vi "Test - Engine.vi"(8 "error in (no error)":errorcluster) -> (0 "error out":errorcluster)   [LabVIEW 2017]
uses:
  Controls/Test - Driver control.ctl
  Controls/RT- Queue States.ctl
  <vilib>/Utility/file.llb/Read Delimited Spreadsheet (string).vi
  Test - Step config.ctl
  Test - Message cluster.ctl
  SubVIs/SubVI - Global.vi
  <vilib>/Platform/TimedLoop/XDataNode/XDataNode.xnode
  <vilib>/Platform/TimedLoop/XDataNode/nitl_modes.ctl
  <vilib>/Platform/TimedLoop/XDataNode/XDNodeRunTimeDep.lvlib
  <vilib>/Platform/TimedLoop/XDataNode/wakeup.ctl
  <vilib>/Platform/TimedLoop/XDataNode/timing_clust.ctl
  Test - Step Result.ctl
  Controls/RT- Get Set.ctl
  DataLog/Datalog -Driver Control.ctl
  DAQ/DAQ -Driver Control.ctl
  Controls/TCP - Driver Control.ctl
  Controls/TCP - Signal Names.ctl
  Controls/TCP - Signals.ctl
  Controls/Dyno Config Driver.ctl
  SubVIs/Get - Set.ctl
panel:
  out "appended array":T1[](array[typedef])
  out "Waveform Chart":dbl(graph)
  out "Results":T2[](array[typedef])
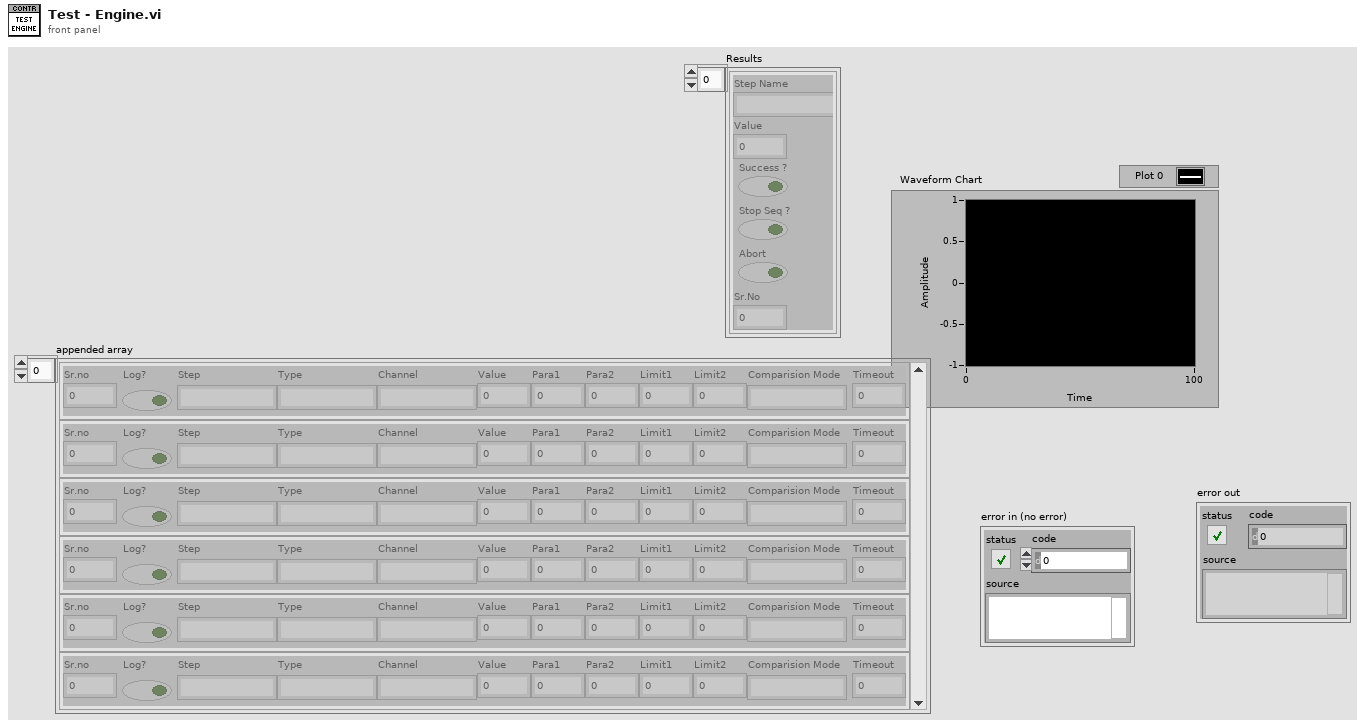
[diagram p1: front panel]
types:
  T1 = typedef "Test - Step config.ctl" = cluster{"Sr.no":i32, "Log?":bool, "Step":string, "Type":string, "Channel":string, "Value":dbl, "Para1":dbl, "Para2":dbl, "Limit1":dbl, "Limit2":dbl, "Comparision Mode":string, "Timeout":dbl}
  T2 = typedef "Test - Step Result.ctl" = cluster{"Step Name":string, "Value":dbl, "Success ?":bool, "Stop Seq ?":bool, "Abort":bool, "Sr.No":i32}
  T3 = typedef "Test - Message cluster.ctl" = cluster{"Preslip Sequence":T1[], "Step No":i32, "Step Value":T1, "Slip Parameter":T1[], "Slip Timer":dbl, "Postslip Sequence":T1[], "Postslip ?":bool, "Step Result":T2}
  T4 = typedef "Test - Driver control.ctl" = enum16{"Init", "Load Sequence File", "Test Running", "Index Step", "Execute Step", "Send Results", "Sequence Complete", "Sequence Aborted", "Stop Sequence Triggered", "Update Manual Values", "Start Aux Logging", "Stop Aux Logging", "Change Dyno Selection", "Reset Emergency Fault", "Get Dyno Config", "Exit"}
  T5 = typedef "RT- Queue States.ctl" = enum16{"Initialize", "Enqueue", "Enqueue Priority", "Dequeue", "Flush", "Destroy"}
  T6 = typedef "Dyno Config Driver.ctl" = enum16{"Read File", "Set", "Get", "Write File", "Set Temp Value"}
  T7 = typedef "Get - Set.ctl" = enum16{"SET", "GET", "Derived"}
  T8 = typedef "TCP - Driver Control.ctl" = enum16{"Download Config Files", "Test Started", "Test Running", "Update Sensor Data", "Test Complete"}
  T9 = typedef "TCP - Signal Names.ctl" = enum16{"Test Running", "Update Sensor Data", "Start Test", "Test Started", "Sequence Complete", "Seuence Aborted", "Abort Test", "Test Settings Updated", "Log Path", "Start Aux Logging", "Stop Aux Logging", "Reset Emergency", "Copy Log File", "Generate Alarm", "Download Files", "Send Test Details"}
  T10 = typedef "TCP - Signals.ctl" = cluster{"Signal":T9, "Value":bool, "Data":variant}
  T11 = typedef "RT- Get Set.ctl" = enum16{"Reset", "Get", "Set"}
  T12 = typedef "Datalog -Driver Control.ctl" = enum16{"Timeout", "Init", "Create Date Folder", "Create File", "Log Data", "Close File", "Update Fileinfo", "Download Files from Windows", "Exit"}
  T13 = typedef "DAQ -Driver Control.ctl" = enum16{"Timeout", "Init", "Config FPGA", "Start Acquisition", "Read Data", "Stop Acquisition", "Flush Queue", "Exit"}
  T14 = typedef "XDNodeRunTimeDep.lvlib/timing_clust.ctl" = cluster{"Expected End [f-1]":u64, "Actual End [f-1]":u64, "Finished Late? [f-1]":bool, "Expected End [i-1]":u64, "Actual End [i-1]":u64, "Finished Late? [i-1]":bool, "Expected Start [i]":u64, "Actual Start [i]":u64, "Expected Start [f]":u64, "Actual Start [f]":u64, "Source Name":string, "Structure Name":string, "Period":i64, "Deadline":i64, "Offset":i64, "Start":i64, "Priority":i32, "Timeout":i32, "Mode":T15, "Wakeup Reason":T16, "Error":errorcluster, "Source Type":string, "Secondary Source Type":string, "Global End Time":u64, "Global Start Time":u64, "Frame Duration":u64, "Iteration Duration":u64, "Assigned CPU":i32, "I/O Scan Engine Mode":u32}
  T15 = typedef "XDNodeRunTimeDep.lvlib/nitl_modes.ctl" = enum32{"No Change", "Process missed periods, maintain original phase", "Discard missed periods, maintain original phase", "Process missed periods, ignore original phase", "Discard missed periods, ignore original phase"}
  T16 = typedef "XDNodeRunTimeDep.lvlib/wakeup.ctl" = enum32{"Normal", "Aborted", "Asynchronous wakeup", "Timing source error", "Timed loop error", "Timeout"}
  T17 = typedef "TCP - Driver Control.ctl" = enum16{"Test Settings", "Boolean Commands", "Test Results"}
  T18 = typedef "TCP - Signal Names.ctl" = enum16{"Start Test", "Test Started", "Sequence Complete", "Seuence Aborted", "Abort Test", "Test Settings Updated", "Log Path", "Update Manual Values", "Start Aux Logging", "Aux Log Started", "Stop Aux Logging", "Aux Log Stopped", "Set Dyno Config", "Get PID Values", "Reset Emergency", "Copy Log File", "Download Files"}
  T19 = cluster{"proportional gain (Kc)":dbl, "integral time (Ti, min)":dbl, "derivative time (Td, min)":dbl}
  T20 = typedef "RT- Dyno Parameters.ctl" = cluster{"PID gains":cluster{"proportional gain (Kc)":dbl, "integral time (Ti, min)":dbl, "derivative time (Td, min)":dbl}, "Channel No":i32, "Dyno Type":string}
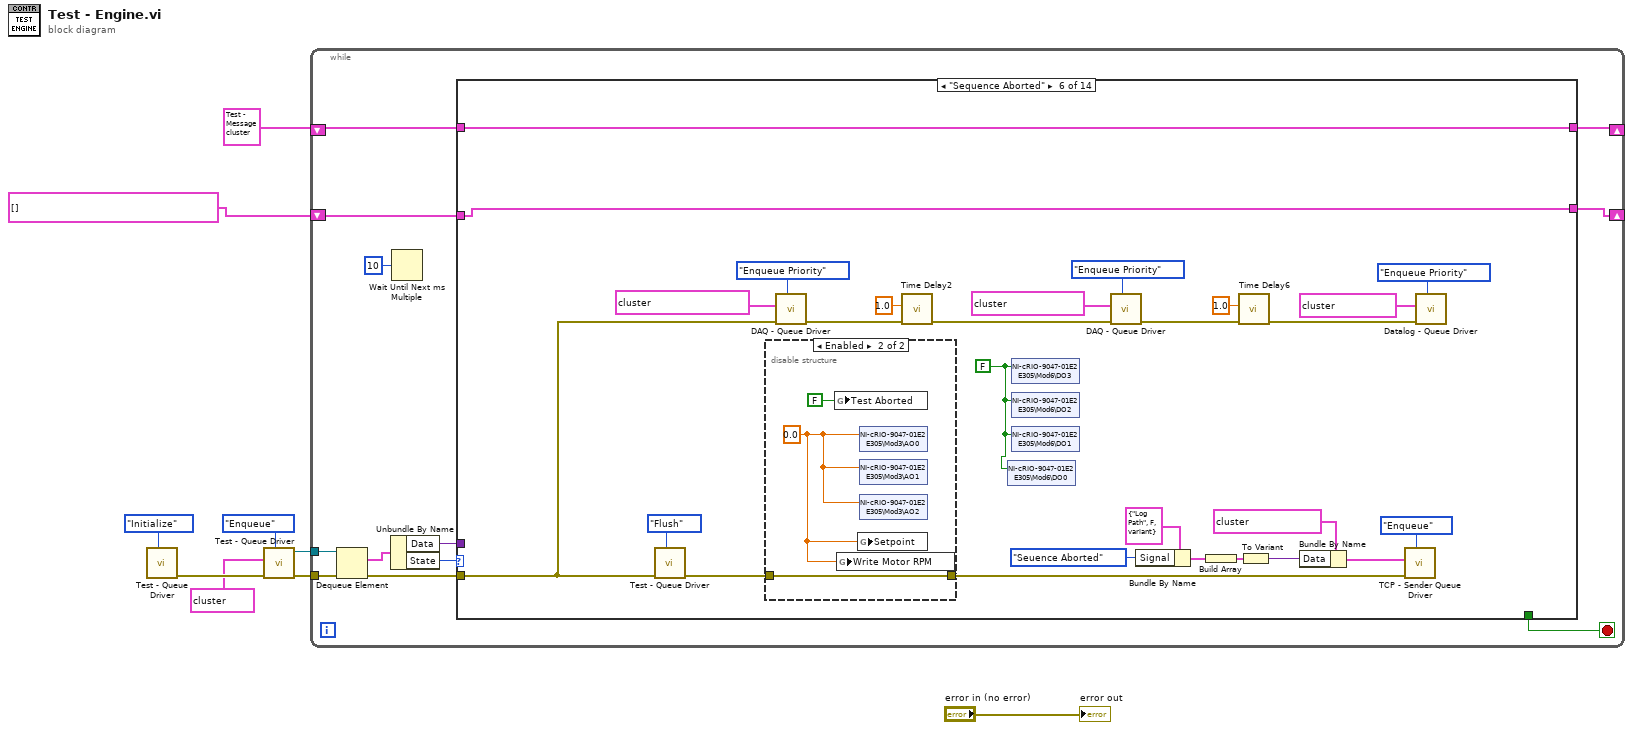
[diagram p0: block diagram]
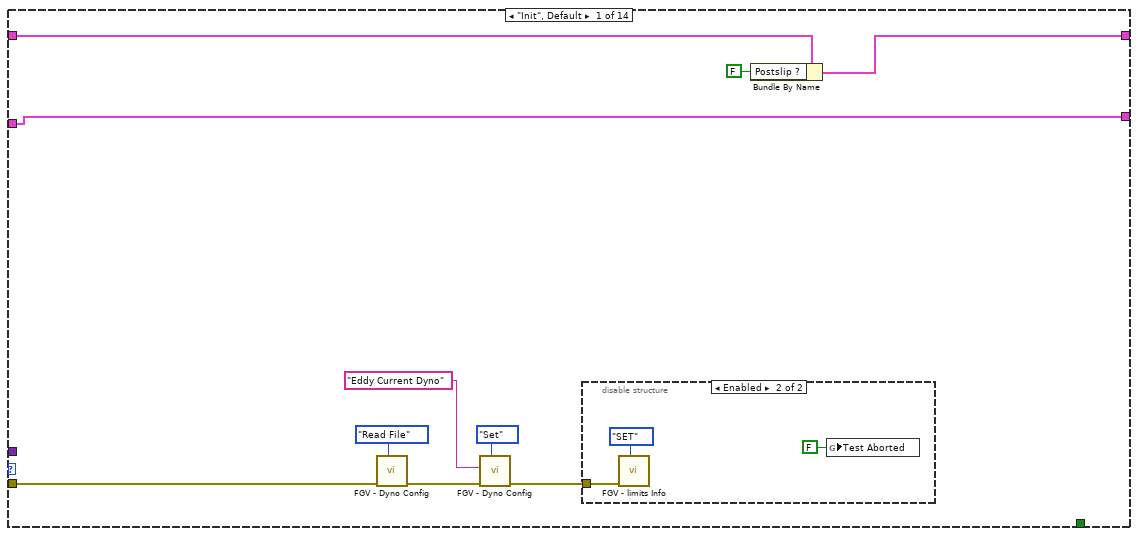
[diagram p2: hidden frame]
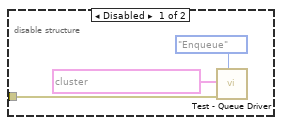
[diagram p3: hidden frame]
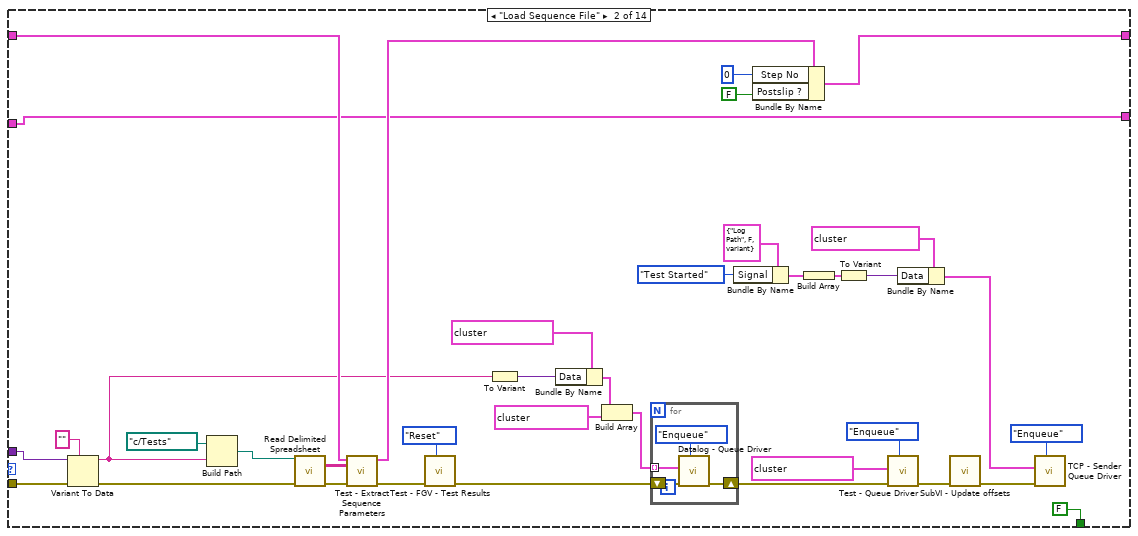
[diagram p4: hidden frame]
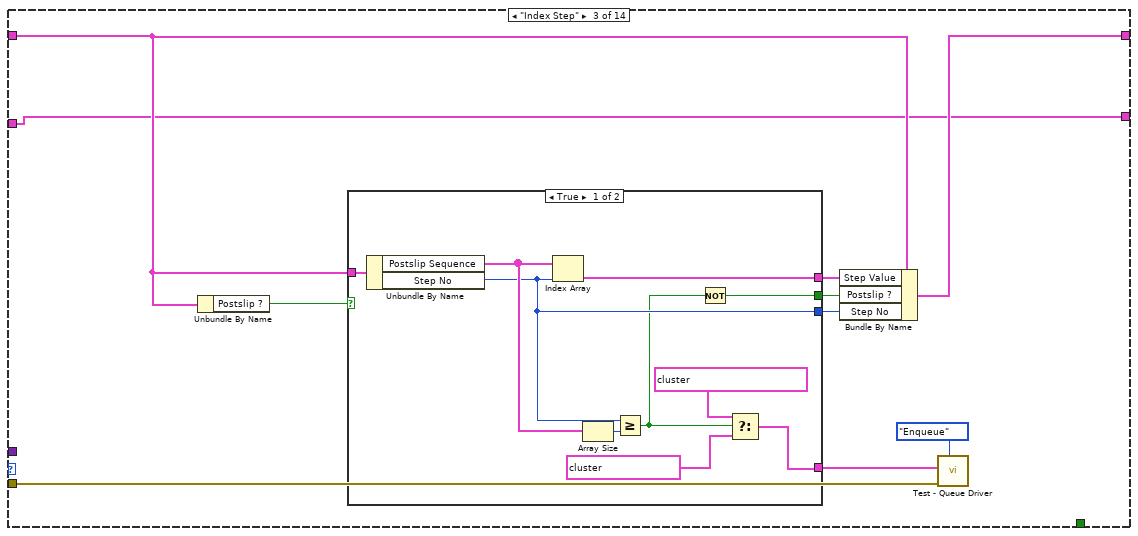
[diagram p5: hidden frame]
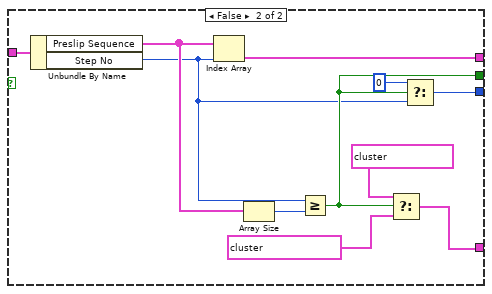
[diagram p6: hidden frame]
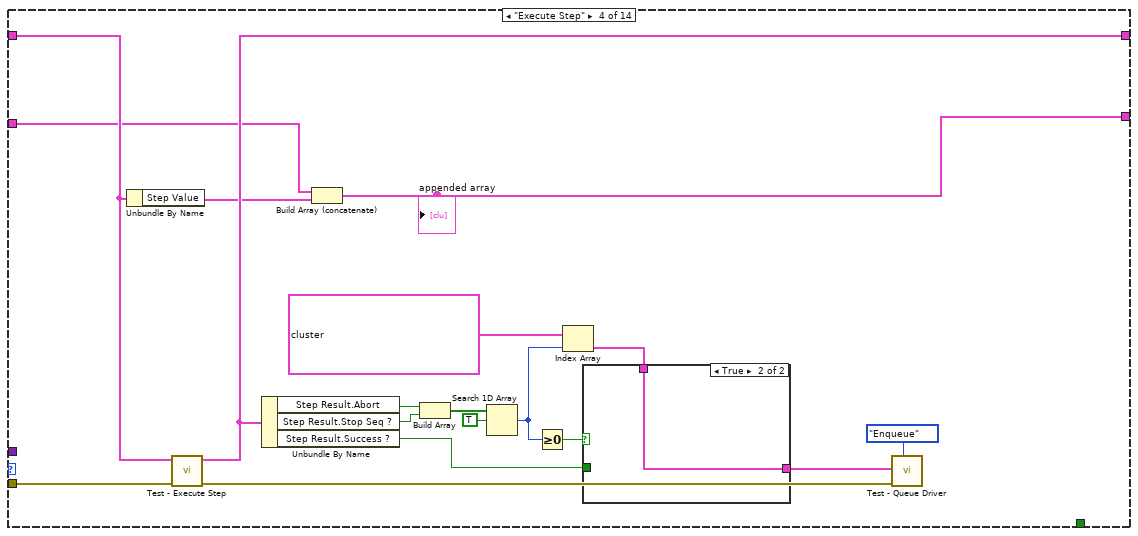
[diagram p7: hidden frame]
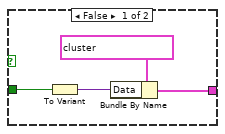
[diagram p8: hidden frame]
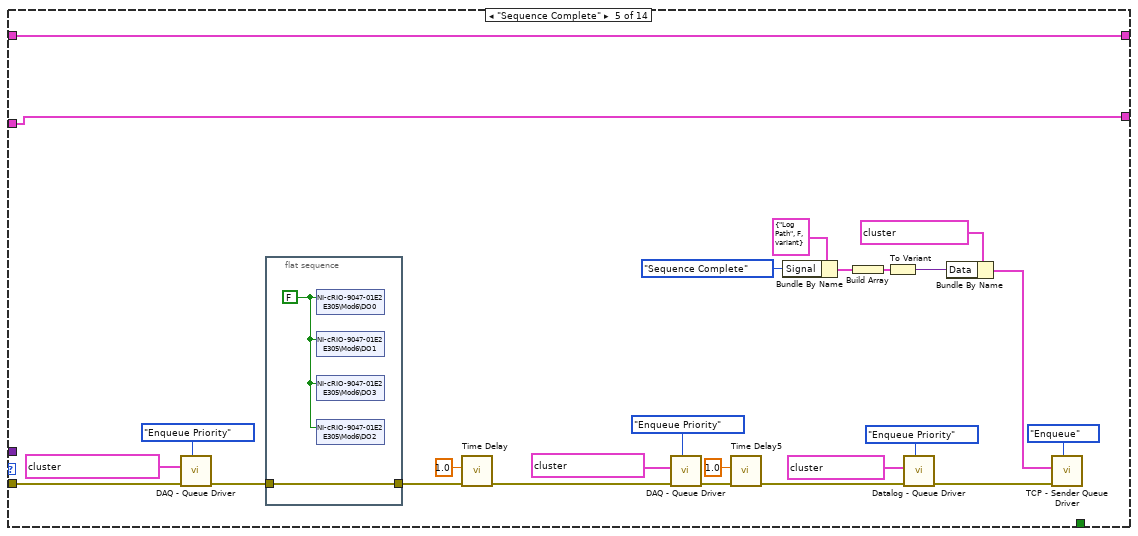
[diagram p9: hidden frame]
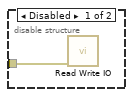
[diagram p10: hidden frame]
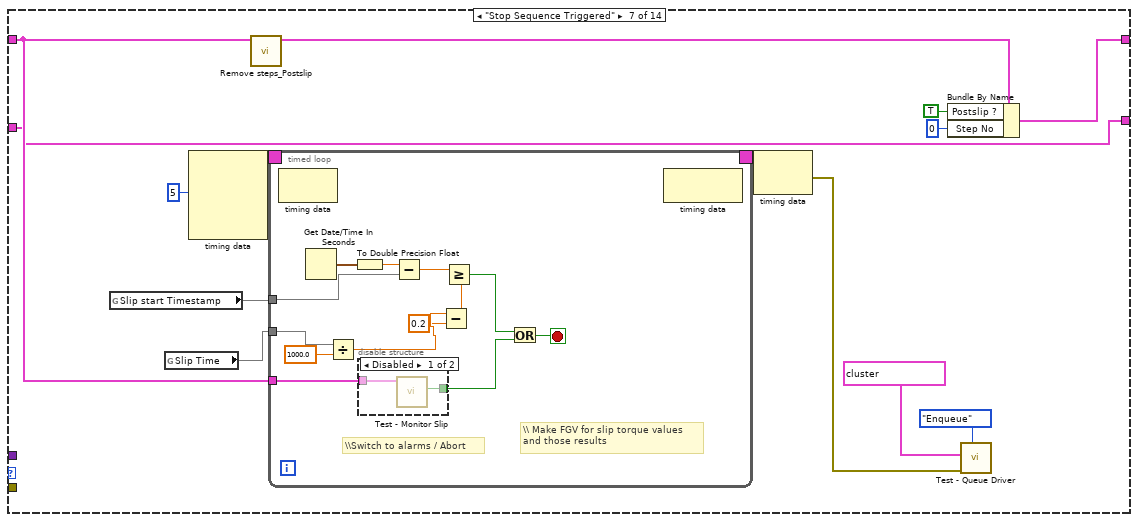
[diagram p11: hidden frame]
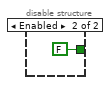
[diagram p12: hidden frame]
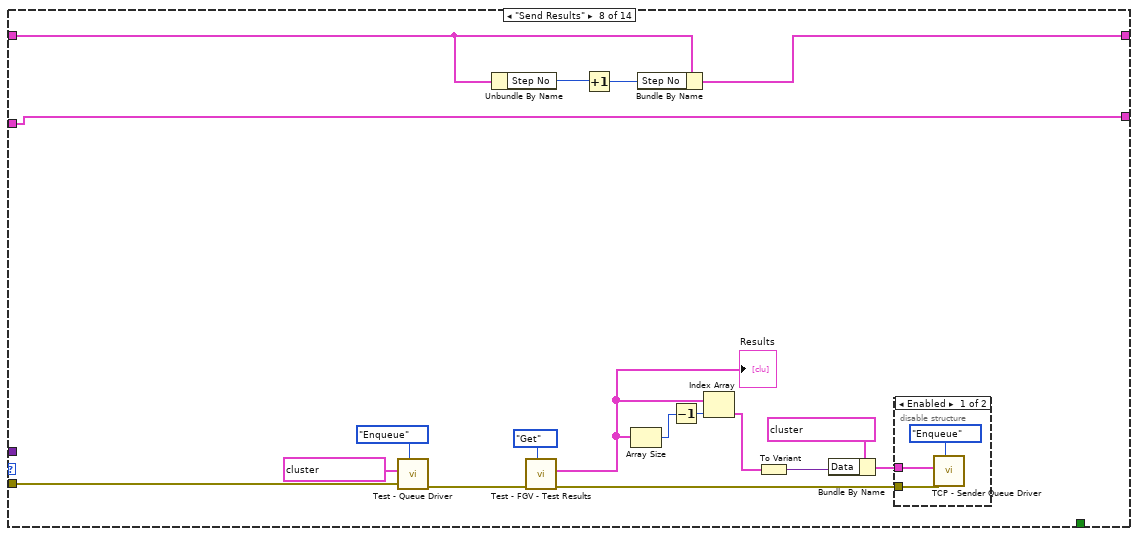
[diagram p13: hidden frame]
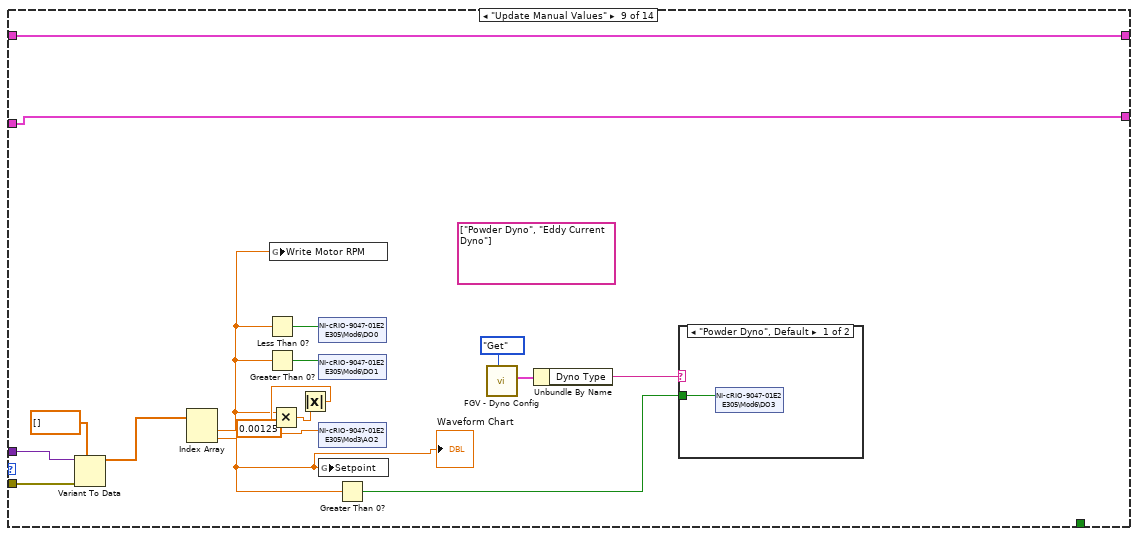
[diagram p15: hidden frame]
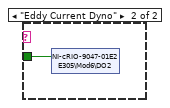
[diagram p16: hidden frame]
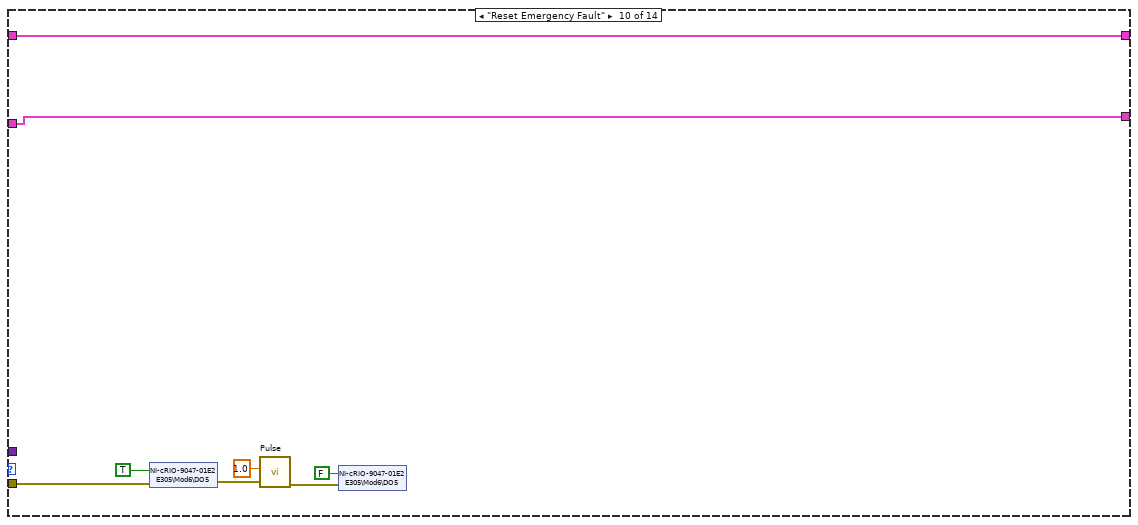
[diagram p17: hidden frame]
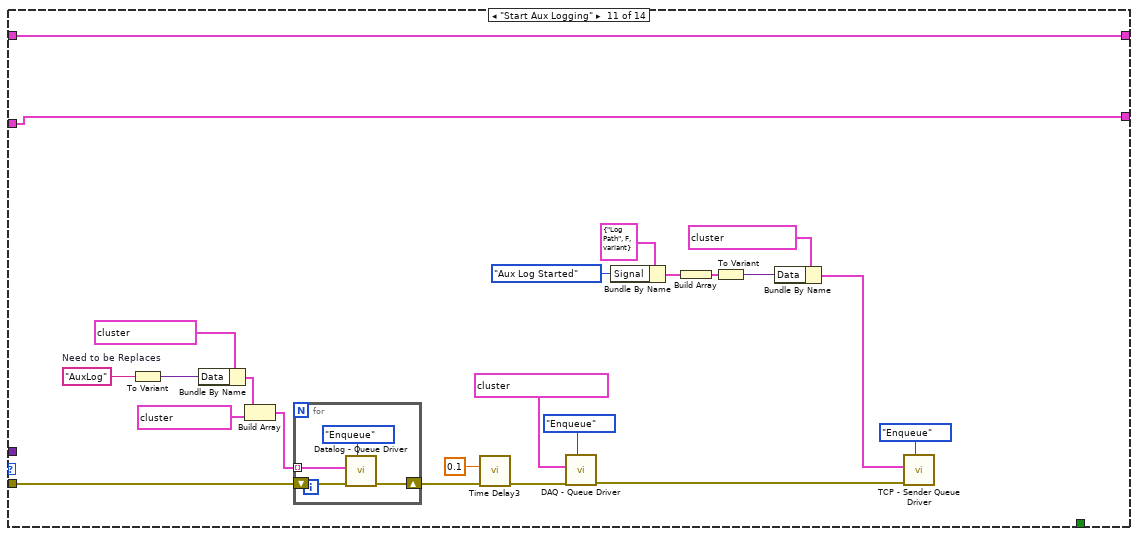
[diagram p18: hidden frame]
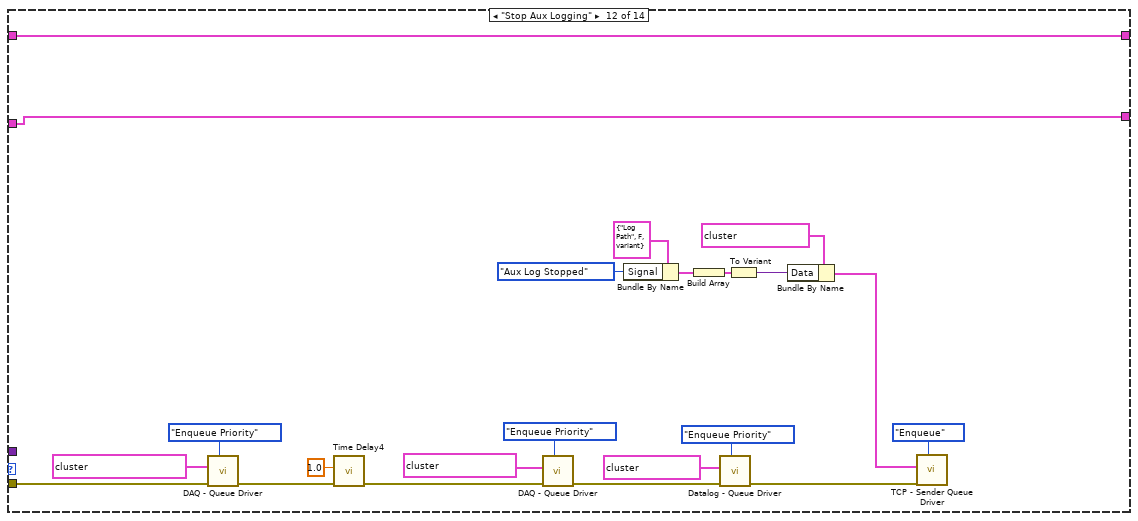
[diagram p19: hidden frame]
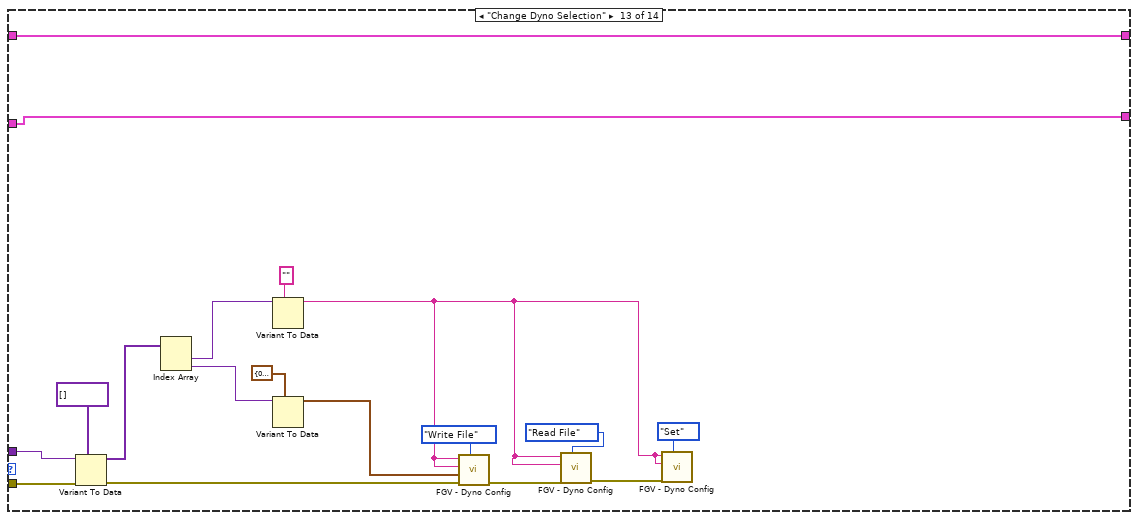
[diagram p20: hidden frame]
diagram:
  n1 = call "Test - Queue Driver.vi"("Cases"=RT-_Queue_States."Initialize") -> ("error out"=w7:errorcluster)  [unwired: 8 in, 2 out]
  n2 = call "Test - Queue Driver.vi"("Cases"=RT-_Queue_States."Enqueue", "error in (no error)"=w7, "Element In"=cluster{"Data":variant, "State":T4} {"Data"=variant, "State"=enum."Init"}) -> ("error out"=w5:errorcluster, "queue out"=w4:refnum<queue>)  [unwired: 6 in, 1 out]
  n3 = while {
    tunnel: w5 -> [w21]
    tunnel: w4 -> [w20]
    shift-right: [w13] -> _
    shift-left: T3 {"Preslip Sequence"=[], "Step No"=0, "Step Value"={"Sr.no"=0, "Log?"=FALSE, "Step"="", "Type"="", "Channel"="", "Value"=0.0, "Para1"=0.0, "Para2"=0.0, "Limit1"=0.0, "Limit2"=0.0, "Comparision Mode"="", "Timeout"=0.0}, "Slip Parameter"=[], "Slip Timer"=0.0, "Postslip Sequence"=[], "Postslip ?"=FALSE, "Step Result"={"Step Name"="", "Value"=0.0, "Success ?"=TRUE, "Stop Seq ?"=TRUE, "Abort"=TRUE, "Sr.No"=0}} -> [w12]
    shift-right: [w10] -> _
    shift-left: T1[] [] ("element") -> [w11]
    stop <- w14 stop-if-true
    n4 = Dequeue Element(queue=w20, error in (no error)=w21) -> (element=w19:cluster{"Data":variant, "State":T4}, error out=w18:errorcluster)  [unwired: 1 in, 2 out]
    n5 = Unbundle By Name(w19) -> ("Data"=w16:variant, "State"=w17:T4)
    n6 = Wait Until Next ms Multiple(millisecond multiple=u32 10) -> ()  [unwired: 1 out]
    n7 = case shown="\"Sequence Aborted\"" w17 {
      tunnel: w18 -> [w27 w53 w85 w127 w152 w175 _ w239 w264 w269 w291 w319 w340 w360]
      tunnel: w16 -> [_ w55 _ _ _ _ _ _ w263 _ _ _ w339 w358]
      tunnel: [_ FALSE _ _ _ _ _ _ _ _ _ _ _ _] -> w14
      tunnel: w12 -> [w30 w73 w83 w113 w157 w186 w193 w243 w265 w275 w298 w324 w342 w363]
      tunnel: [w29 w66 w87 w117 w157 w186 w199 w242 w265 w275 w298 w324 w342 w363] -> w13
      tunnel: w11 -> [w22 w38 w79 w111 w135 w161 w191 w228 w249 w268 w276 w303 w325 w343]
      tunnel: [w22 w38 w79 w110 w135 w161 w191 w228 w249 w268 w276 w303 w325 w343] -> w10
      frame "Init", Default {
        n8 = call "FGV - Dyno Config.vi"("Control"=Dyno_Config_Driver."Read File", "error in (no error)"=w27) -> ("error out"=w25:errorcluster)  [unwired: 8 in, 1 out]
        n9 = call "FGV - Dyno Config.vi"("Control"=Dyno_Config_Driver."Set", "error in (no error)"=w25, "Dyno"="Eddy Current Dyno") -> ("error out"=w24:errorcluster)  [unwired: 7 in, 1 out]
        n10 = disable-structure shown="Enabled" {
          disable-tunnel: w24 -> [w32 w35]
          frame Disabled {
            n11 = call "Test - Queue Driver.vi"("Cases"=RT-_Queue_States."Enqueue", "error in (no error)"=w32, "Element In"=cluster{"Data":variant, "State":T4} {"Data"=variant, "State"=enum."Load Sequence File"}) -> ()  [unwired: 6 in, 3 out]
          }
          frame Enabled {
            n12 = call "FGV - limits Info.vi"("GET/SET"=Get_-_Set."SET", "error in (no error)"=w35) -> ()  [unwired: 8 in, 2 out]
            n13 = global write "SubVI - Global.vi" "Test Aborted"(FALSE ("Test Aborted")) -> ()
          }
        }
        n14 = Bundle By Name(cluster=w30, "Postslip ?"=FALSE) -> (w29:T3)
      }
      frame "Load Sequence File" {
        n15 = Variant To Data(error in=w53, type="", Variant=w55) -> (data=w41:string, error out=w52:errorcluster)
        n16 = Build Path(base path=path "c:/Tests" ("file path (dialog if empty)"), name or relative path=w41) -> (appended path=w50:path)
        n17 = call-poly <vilib>:"Read Delimited Spreadsheet.vi"("file path (dialog if empty)"=w50, "error in (no error)"=w52) -> ("all rows"=w72:string[][], "error out"=w71:errorcluster)  [unwired: 8 in, 4 out]
        n18 = call "Test - Extract Sequence Parameters.vi"("error in (no error)"=w71, "Sequence Data"=w72, "Cluster in"=w73) -> ("error out"=w57:errorcluster, "output cluster"=w67:T3)  [unwired: 7 in]
        n19 = call "Test - FGV - Test Results.vi"("Get/Set"=RT-_Get_Set."Reset", "error in (no error)"=w57) -> ("error out"=w56:errorcluster)  [unwired: 8 in, 1 out]
        n20 = To Variant(anything=w41) -> (Variant=w64:variant)
        n21 = Bundle By Name(cluster=cluster{"Data":variant, "State":T12} {"Data"=variant, "State"=enum."Create File"} ("Element In"), "Data"=w64) -> (w60:cluster{"Data":variant, "State":T12})
        n22 = Build Array(w60, cluster{"Data":variant, "State":T12} {"Data"=variant, "State"=enum."Log Data"} ("element")) -> (w59:cluster{"Data":variant, "State":T12}[])
        n23 = for {
          tunnel: w59 -> [w75] mode=indexing
          shift-right: [w76] -> w62
          shift-left: w56 -> [w77]
          n24 = call "Datalog - Queue Driver.vi"("Cases"=RT-_Queue_States."Enqueue", "error in (no error)"=w77, "Element In"=w75) -> ("error out"=w76:errorcluster)  [unwired: 6 in, 2 out]
        }
        n25 = Bundle By Name(cluster=T10 {"Signal"=enum."Log Path", "Value"=FALSE, "Data"=variant}, "Signal"=TCP_-_Signal_Names."Test Started") -> (w46:T10)
        n26 = Bundle By Name(cluster=w67, "Step No"=0, "Postslip ?"=FALSE) -> (w66:T3)
        n27 = Build Array(w46) -> (w44:T10[])
        n28 = To Variant(anything=w44) -> (Variant=w43:variant)
        n29 = call "Test - Queue Driver.vi"("Cases"=RT-_Queue_States."Enqueue", "error in (no error)"=w62, "Element In"=cluster{"Data":variant, "State":T4} {"Data"=variant, "State"=enum."Index Step"}) -> ("error out"=w40:errorcluster)  [unwired: 6 in, 2 out]
        n30 = Bundle By Name(cluster=cluster{"Data":variant, "State":T8} {"Data"=variant, "State"=enum."Test Started"} ("Element In"), "Data"=w43) -> (w42:cluster{"Data":variant, "State":T8})
        n31 = call "SubVI - Update offsets.vi"("error in (no error)"=w40) -> ("error out"=w39:errorcluster)  [unwired: 10 in]
        n32 = call "TCP - Sender Queue Driver.vi"("Cases"=RT-_Queue_States."Enqueue", "error in (no error)"=w39, "Element In"=w42) -> ()  [unwired: 6 in, 3 out]
      }
      frame "Index Step" {
        n33 = Unbundle By Name(w83) -> ("Postslip ?"=w82:bool)
        n34 = case shown="True" w82 {
          tunnel: [w98 w103] -> w88
          tunnel: [w94 w106] -> w84
          tunnel: w83 -> [w93 w105]
          tunnel: [w89 w102] -> w81
          tunnel: [w91 w99] -> w80
          frame True {
            n35 = Unbundle By Name(w93) -> ("Postslip Sequence"=w97:T1[], "Step No"=w91:i32)
            n36 = Index Array(array=w97, index=w91) -> (element=w98:T1)
            n37 = Array Size(array=w97) -> (size(s)=w92:i32)
            n38 = Greater Or Equal?(x=w91, y=w92) -> (x >= y?=w90:bool)
            n39 = Not(x=w90) -> (.not. x?=w89:bool)
            n40 = Select(t=cluster{"Data":variant, "State":T4} {"Data"=variant, "State"=enum."Sequence Complete"} ("Element In"), s=w90, f=cluster{"Data":variant, "State":T4} {"Data"=variant, "State"=enum."Execute Step"} ("Element In")) -> (s? t:f=w94:cluster{"Data":variant, "State":T4})
          }
          frame False {
            n41 = Unbundle By Name(w105) -> ("Preslip Sequence"=w109:T1[], "Step No"=w100:i32)
            n42 = Index Array(array=w109, index=w100) -> (element=w103:T1)
            n43 = Array Size(array=w109) -> (size(s)=w104:i32)
            n44 = Greater Or Equal?(x=w100, y=w104) -> (x >= y?=w102:bool)
            n45 = Select(t=cluster{"Data":variant, "State":T4} {"Data"=variant, "State"=enum."Index Step"} ("Element In"), s=w102, f=cluster{"Data":variant, "State":T4} {"Data"=variant, "State"=enum."Execute Step"} ("Element In")) -> (s? t:f=w106:cluster{"Data":variant, "State":T4})
            n46 = Select(t=0 ("Step No"), s=w102, f=w100) -> (s? t:f=w99:i32)
          }
        }
        n47 = Bundle By Name(cluster=w83, "Step Value"=w88, "Postslip ?"=w81, "Step No"=w80) -> (w87:T3)
        n48 = call "Test - Queue Driver.vi"("Cases"=RT-_Queue_States."Enqueue", "error in (no error)"=w85, "Element In"=w84) -> ()  [unwired: 6 in, 3 out]
      }
      frame "Execute Step" {
        n49 = Unbundle By Name(w113) -> ("Step Value"=w112:T1)
        n50 = call "Test - Execute Step.vi"("error in (no error)"=w127, "Cluster"=w113) -> ("error out"=w125:errorcluster, "output cluster"=w117:T3)  [unwired: 8 in]
        n51 = Unbundle By Name(w117) -> ("Step Result.Abort"=w116:bool, "Step Result.Stop Seq ?"=w115:bool, "Step Result.Success ?"=w114:bool)
        n52 = Build Array (concatenate)(w111, w112) -> (w110:T1[])
        "appended array" <- w110
        n53 = Build Array(w116, w115) -> (w123:bool[])
        n54 = Search 1D Array(1D array=w123, element=TRUE) -> (index of element=w120:i32)  [unwired: 1 in]
        n55 = Greater Or Equal To 0?(x=w120) -> (x >= 0?=w119:bool)
        n56 = Index Array(array=cluster{"Data":variant, "State":T4}[] [{"Data"=variant, "State"=enum."Sequence Aborted"}, {"Data"=variant, "State"=enum."Stop Sequence Triggered"}], index=w120) -> (element=w118:cluster{"Data":variant, "State":T4})
        n57 = case shown="True" w119 {
          tunnel: [w129 w132] -> w124
          tunnel: w114 -> [w128 _]
          tunnel: w118 -> [_ w132]
          frame False {
            n58 = To Variant(anything=w128) -> (Variant=w130:variant)
            n59 = Bundle By Name(cluster=cluster{"Data":variant, "State":T4} {"Data"=variant, "State"=enum."Send Results"} ("Element In"), "Data"=w130) -> (w129:cluster{"Data":variant, "State":T4})
          }
          frame True {
          }
        }
        n60 = call "Test - Queue Driver.vi"("Cases"=RT-_Queue_States."Enqueue", "error in (no error)"=w125, "Element In"=w124) -> ()  [unwired: 6 in, 3 out]
      }
      frame "Sequence Complete" {
        n61 = call "DAQ - Queue Driver.vi"("Cases"=RT-_Queue_States."Enqueue Priority", "error in (no error)"=w152, "Element In"=cluster{"Data":variant, "States":T13} {"Data"=variant, "States"=enum."Stop Acquisition"}) -> ("error out"=w134:errorcluster)  [unwired: 6 in, 2 out]
        n62 = flat-sequence {
          tunnel: [w159] -> w133
          tunnel: w134 -> [w159]
          frame #0 {
            w158 = FALSE ("DO0")
            n63 = shared-variable "NI-cRIO-9047-01E2E305\\Mod6\\DO0"(w158) -> ()  [unwired: 1 in, 1 out]
            n64 = shared-variable "NI-cRIO-9047-01E2E305\\Mod6\\DO1"(w158) -> ()  [unwired: 1 in, 1 out]
            n65 = shared-variable "NI-cRIO-9047-01E2E305\\Mod6\\DO3"(w158) -> ()  [unwired: 1 in, 1 out]
            n66 = shared-variable "NI-cRIO-9047-01E2E305\\Mod6\\DO2"(w158) -> ()  [unwired: 1 in, 1 out]
          }
        }
        n67 = call "Time Delay"("error in (no error)"=w133, "Delay Time (s)"=1.0) -> ("error out"=w148:errorcluster)  [unwired: 9 in]
        n68 = call "DAQ - Queue Driver.vi"("Cases"=RT-_Queue_States."Enqueue Priority", "error in (no error)"=w148, "Element In"=cluster{"Data":variant, "States":T13} {"Data"=variant, "States"=enum."Flush Queue"}) -> ("error out"=w137:errorcluster)  [unwired: 6 in, 2 out]
        n69 = call "Time Delay5"("error in (no error)"=w137, "Delay Time (s)"=1.0) -> ("error out"=w136:errorcluster)  [unwired: 9 in]
        n70 = Bundle By Name(cluster=T10 {"Signal"=enum."Log Path", "Value"=FALSE, "Data"=variant}, "Signal"=TCP_-_Signal_Names."Sequence Complete") -> (w144:T10)
        n71 = Build Array(w144) -> (w142:T10[])
        n72 = To Variant(anything=w142) -> (Variant=w141:variant)
        n73 = call "Datalog - Queue Driver.vi"("Cases"=RT-_Queue_States."Enqueue Priority", "error in (no error)"=w136, "Element In"=cluster{"Data":variant, "State":T12} {"Data"=variant, "State"=enum."Close File"}) -> ("error out"=w139:errorcluster)  [unwired: 6 in, 2 out]
        n74 = Bundle By Name(cluster=cluster{"Data":variant, "State":T8} {"Data"=variant, "State"=enum."Test Started"} ("Element In"), "Data"=w141) -> (w140:cluster{"Data":variant, "State":T8})
        n75 = call "TCP - Sender Queue Driver.vi"("Cases"=RT-_Queue_States."Enqueue", "error in (no error)"=w139, "Element In"=w140) -> ()  [unwired: 6 in, 3 out]
      }
      frame "Sequence Aborted" {
        w160 = FALSE ("DO3")
        n76 = call "Test - Queue Driver.vi"("Cases"=RT-_Queue_States."Flush", "error in (no error)"=w175) -> ("error out"=w174:errorcluster)  [unwired: 7 in, 2 out]
        n77 = disable-structure shown="Enabled" {
          disable-tunnel: w174 -> [w187 w190]
          disable-tunnel: [_ w190] -> w165
          frame Disabled {
            n78 = call "Read Write IO.vi"("Error in"=w187) -> ()  [unwired: 12 in, 3 out]
          }
          frame Enabled {
            w188 = 0.0 ("AO0")
            n79 = global write "SubVI - Global.vi" "Test Aborted"(FALSE ("Test Aborted")) -> ()
            n80 = global write "SubVI - Global.vi" "Write Motor RPM"(w188) -> ()
            n81 = global write "SubVI - Global.vi" "Setpoint"(w188) -> ()
            n82 = shared-variable "NI-cRIO-9047-01E2E305\\Mod3\\AO0"(w188) -> ()  [unwired: 1 in, 1 out]
            n83 = shared-variable "NI-cRIO-9047-01E2E305\\Mod3\\AO1"(w188) -> ()  [unwired: 1 in, 1 out]
            n84 = shared-variable "NI-cRIO-9047-01E2E305\\Mod3\\AO2"(w188) -> ()  [unwired: 1 in, 1 out]
          }
        }
        n85 = call "DAQ - Queue Driver.vi"("Cases"=RT-_Queue_States."Enqueue Priority", "error in (no error)"=w175, "Element In"=cluster{"Data":variant, "States":T13} {"Data"=variant, "States"=enum."Stop Acquisition"}) -> ("error out"=w179:errorcluster)  [unwired: 6 in, 2 out]
        n86 = call "Time Delay2"("error in (no error)"=w179, "Delay Time (s)"=1.0) -> ("error out"=w178:errorcluster)  [unwired: 9 in]
        n87 = shared-variable "NI-cRIO-9047-01E2E305\\Mod6\\DO0"(w160) -> ()  [unwired: 1 in, 1 out]
        n88 = shared-variable "NI-cRIO-9047-01E2E305\\Mod6\\DO3"(w160) -> ()  [unwired: 1 in, 1 out]
        n89 = shared-variable "NI-cRIO-9047-01E2E305\\Mod6\\DO2"(w160) -> ()  [unwired: 1 in, 1 out]
        n90 = shared-variable "NI-cRIO-9047-01E2E305\\Mod6\\DO1"(w160) -> ()  [unwired: 1 in, 1 out]
        n91 = call "DAQ - Queue Driver.vi"("Cases"=RT-_Queue_States."Enqueue Priority", "error in (no error)"=w178, "Element In"=cluster{"Data":variant, "States":T13} {"Data"=variant, "States"=enum."Flush Queue"}) -> ("error out"=w163:errorcluster)  [unwired: 6 in, 2 out]
        n92 = Bundle By Name(cluster=T10 {"Signal"=enum."Log Path", "Value"=FALSE, "Data"=variant}, "Signal"=TCP_-_Signal_Names."Seuence Aborted") -> (w170:T10)
        n93 = Build Array(w170) -> (w168:T10[])
        n94 = call "Time Delay6"("error in (no error)"=w163, "Delay Time (s)"=1.0) -> ("error out"=w162:errorcluster)  [unwired: 9 in]
        n95 = To Variant(anything=w168) -> (Variant=w167:variant)
        n96 = Bundle By Name(cluster=cluster{"Data":variant, "State":T8} {"Data"=variant, "State"=enum."Test Started"} ("Element In"), "Data"=w167) -> (w166:cluster{"Data":variant, "State":T8})
        n97 = call "TCP - Sender Queue Driver.vi"("Cases"=RT-_Queue_States."Enqueue", "error in (no error)"=w165, "Element In"=w166) -> ()  [unwired: 6 in, 3 out]
        n98 = call "Datalog - Queue Driver.vi"("Cases"=RT-_Queue_States."Enqueue Priority", "error in (no error)"=w162, "Element In"=cluster{"Data":variant, "State":T12} {"Data"=variant, "State"=enum."Close File"}) -> ()  [unwired: 6 in, 3 out]
      }
      frame "Stop Sequence Triggered" {
        n99 = global read "SubVI - Global.vi" "Slip start Timestamp"() -> (w201)
        n100 = global read "SubVI - Global.vi" "Slip Time"() -> (w194)
        n101 = node-c288(i64 5 ("Period")) -> (w204:T14)  [unwired: 3 in]
        n102 = call "Remove steps_Postslip.vi"("Cluster"=w193) -> ("output cluster"=w192:T3)  [unwired: 10 in]
        n103 = timed-loop {
          timing: w204 -> [_]
          timing-out: [_] -> w203
          tunnel: w201 -> [w214]
          tunnel: w194 -> [w208]
          tunnel: w193 -> [w213]
          stop <- w210 stop-if-true
          # "\\\\ Make FGV for slip torque values\nand those results"
          # "\\\\Switch to alarms / Abort"
          n104 = node-c288() -> ()  [unwired: 1 in, 1 out]
          n105 = Get Date/Time In Seconds() -> (seconds since 1Jan1904=w217:timestamp)
          n106 = Divide(x=w208, y=1000.0) -> (x/y=w206:dbl)
          n107 = To Double Precision Float(number=w217) -> (double precision float=w216:dbl)
          n108 = disable-structure shown="Disabled" {
            disable-tunnel: w213 -> [w219 _]
            disable-tunnel: [w218 FALSE ("Slip Occured ?")] -> w212
            frame Disabled {
              n109 = call "Test - Monitor Slip.vi"("Cluster"=w219) -> ("Slip Occured ?"=w218:bool)  [unwired: 9 in, 1 out]
            }
            frame Enabled {
            }
          }
          n110 = Subtract(x=w216, y=w214) -> (x-y=w215:dbl)
          n111 = Subtract(x=w206, y=0.2) -> (x-y=w207:dbl)
          n112 = Greater Or Equal?(x=w215, y=w207) -> (x >= y?=w211:bool)
          n113 = Or(x=w211, y=w212) -> (x .or. y?=w210:bool)
          n114 = node-c288() -> ()  [unwired: 1 in, 1 out]
        }
        n115 = node-c288(w203) -> (w195:errorcluster)
        n116 = Bundle By Name(cluster=w192, "Postslip ?"=TRUE, "Step No"=0) -> (w199:T3)
        n117 = call "Test - Queue Driver.vi"("Cases"=RT-_Queue_States."Enqueue", "error in (no error)"=w195, "Element In"=cluster{"Data":variant, "State":T4} {"Data"=variant, "State"=enum."Index Step"}) -> ()  [unwired: 6 in, 3 out]
      }
      frame "Send Results" {
        n118 = call "Test - Queue Driver.vi"("Cases"=RT-_Queue_States."Enqueue", "error in (no error)"=w239, "Element In"=cluster{"Data":variant, "State":T4} {"Data"=variant, "State"=enum."Index Step"}) -> ("error out"=w238:errorcluster)  [unwired: 6 in, 2 out]
        n119 = Unbundle By Name(w243) -> ("Step No"=w245:i32)
        n120 = call "Test - FGV - Test Results.vi"("Get/Set"=RT-_Get_Set."Get", "error in (no error)"=w238) -> ("error out"=w233:errorcluster, "Results"=w230:T2[])  [unwired: 8 in]
        "Results" <- w230
        n121 = Increment(x=w245) -> (x+1=w244:i32)
        n122 = Array Size(array=w230) -> (size(s)=w232:i32)
        n123 = Bundle By Name(cluster=w243, "Step No"=w244) -> (w242:T3)
        n124 = Decrement(x=w232) -> (x-1=w231:i32)
        n125 = Index Array(array=w230, index=w231) -> (element=w229:T2)
        n126 = To Variant(anything=w229) -> (Variant=w236:variant)
        n127 = Bundle By Name(cluster=cluster{"Data":variant, "State":T17} {"Data"=variant, "State"=enum."Test Results"} ("Element In"), "Data"=w236) -> (w234:cluster{"Data":variant, "State":T17})
        n128 = disable-structure shown="Enabled" {
          disable-tunnel: w234 -> [w247 _]
          disable-tunnel: w233 -> [w246 _]
          frame Enabled {
            n129 = call "TCP - Sender Queue Driver.vi"("Cases"=RT-_Queue_States."Enqueue", "error in (no error)"=w246, "Element In"=w247) -> ()  [unwired: 6 in, 3 out]
          }
          frame Disabled {
          }
        }
      }
      frame "Update Manual Values" {
        (unwired) string[] ["Powder Dyno", "Eddy Current Dyno"]
        n130 = Variant To Data(error in=w264, type=dbl[] [], Variant=w263) -> (data=w261:dbl[])  [unwired: 1 out]
        n131 = Index Array(array=w261) -> (element #1=w250:dbl, element #2=w254:dbl)  [unwired: 2 in]
        "Waveform Chart" <- w254
        n132 = Less Than 0?(x=w250) -> (x < 0?=w253:bool)
        n133 = Greater Than 0?(x=w250) -> (x > 0?=w260:bool)
        n134 = global write "SubVI - Global.vi" "Write Motor RPM"(w250) -> ()
        n135 = Multiply(x=w250, y=0.00125) -> (x*y=w252:dbl)
        n136 = Absolute Value(x=w252) -> (abs(x)=w251:dbl)
        n137 = shared-variable "NI-cRIO-9047-01E2E305\\Mod6\\DO0"(w253) -> ()  [unwired: 1 in, 1 out]
        n138 = shared-variable "NI-cRIO-9047-01E2E305\\Mod6\\DO1"(w260) -> ()  [unwired: 1 in, 1 out]
        n139 = shared-variable "NI-cRIO-9047-01E2E305\\Mod3\\AO2"(w251) -> ()  [unwired: 1 in, 1 out]
        n140 = global write "SubVI - Global.vi" "Setpoint"(w254) -> ()
        n141 = Greater Than 0?(x=w254) -> (x > 0?=w258:bool)
        n142 = call "FGV - Dyno Config.vi"("Control"=Dyno_Config_Driver."Get") -> ("Dyno Parameters"=w256:T20)  [unwired: 9 in, 1 out]
        n143 = Unbundle By Name(w256) -> ("Dyno Type"=w255:string)
        n144 = case shown="\"Powder Dyno\", Default" w255 {
          tunnel: w258 -> [w266 w267]
          frame "Powder Dyno", Default {
            n145 = shared-variable "NI-cRIO-9047-01E2E305\\Mod6\\DO3"(w266) -> ()  [unwired: 1 in, 1 out]
          }
          frame "Eddy Current Dyno" {
            n146 = shared-variable "NI-cRIO-9047-01E2E305\\Mod6\\DO2"(w267) -> ()  [unwired: 1 in, 1 out]
          }
        }
      }
      frame "Reset Emergency Fault" {
        n147 = shared-variable "NI-cRIO-9047-01E2E305\\Mod6\\DO5"(TRUE, error in=w269) -> (error out=w273:errorcluster)
        n148 = call "Pulse"("error in (no error)"=w273, "Delay Time (s)"=1.0) -> ("error out"=w271:errorcluster)  [unwired: 9 in]
        n149 = shared-variable "NI-cRIO-9047-01E2E305\\Mod6\\DO5"(FALSE ("DO0"), error in=w271) -> ()  [unwired: 1 out]
      }
      frame "Start Aux Logging" {
        w295 = "AuxLog"  # Need to be Replaces
        n150 = To Variant(anything=w295) -> (Variant=w297:variant)
        n151 = Bundle By Name(cluster=cluster{"Data":variant, "State":T12} {"Data"=variant, "State"=enum."Create File"} ("Element In"), "Data"=w297) -> (w293:cluster{"Data":variant, "State":T12})
        n152 = Build Array(w293, cluster{"Data":variant, "State":T12} {"Data"=variant, "State"=enum."Log Data"} ("element")) -> (w292:cluster{"Data":variant, "State":T12}[])
        n153 = for {
          tunnel: w292 -> [w299] mode=indexing
          shift-right: [w300] -> w287
          shift-left: w291 -> [w301]
          n154 = call "Datalog - Queue Driver.vi"("Cases"=RT-_Queue_States."Enqueue", "error in (no error)"=w301, "Element In"=w299) -> ("error out"=w300:errorcluster)  [unwired: 6 in, 2 out]
        }
        n155 = call "Time Delay3"("error in (no error)"=w287, "Delay Time (s)"=0.1) -> ("error out"=w286:errorcluster)  [unwired: 9 in]
        n156 = call "DAQ - Queue Driver.vi"("Cases"=RT-_Queue_States."Enqueue", "error in (no error)"=w286, "Element In"=cluster{"Data":variant, "States":T13} {"Data"=variant, "States"=enum."Start Acquisition"}) -> ("error out"=w277:errorcluster)  [unwired: 6 in, 2 out]
        n157 = Bundle By Name(cluster=T10 {"Signal"=enum."Log Path", "Value"=FALSE, "Data"=variant}, "Signal"=TCP_-_Signal_Names."Aux Log Started") -> (w282:T10)
        n158 = Build Array(w282) -> (w280:T10[])
        n159 = To Variant(anything=w280) -> (Variant=w279:variant)
        n160 = Bundle By Name(cluster=cluster{"Data":variant, "State":T8} {"Data"=variant, "State"=enum."Test Started"} ("Element In"), "Data"=w279) -> (w278:cluster{"Data":variant, "State":T8})
        n161 = call "TCP - Sender Queue Driver.vi"("Cases"=RT-_Queue_States."Enqueue", "error in (no error)"=w277, "Element In"=w278) -> ()  [unwired: 6 in, 3 out]
      }
      frame "Stop Aux Logging" {
        n162 = call "DAQ - Queue Driver.vi"("Cases"=RT-_Queue_States."Enqueue Priority", "error in (no error)"=w319, "Element In"=cluster{"Data":variant, "States":T13} {"Data"=variant, "States"=enum."Stop Acquisition"}) -> ("error out"=w314:errorcluster)  [unwired: 6 in, 2 out]
        n163 = call "Time Delay4"("error in (no error)"=w314, "Delay Time (s)"=1.0) -> ("error out"=w313:errorcluster)  [unwired: 9 in]
        n164 = call "DAQ - Queue Driver.vi"("Cases"=RT-_Queue_States."Enqueue Priority", "error in (no error)"=w313, "Element In"=cluster{"Data":variant, "States":T13} {"Data"=variant, "States"=enum."Flush Queue"}) -> ("error out"=w316:errorcluster)  [unwired: 6 in, 2 out]
        n165 = Bundle By Name(cluster=T10 {"Signal"=enum."Log Path", "Value"=FALSE, "Data"=variant}, "Signal"=TCP_-_Signal_Names."Aux Log Stopped") -> (w309:T10)
        n166 = Build Array(w309) -> (w307:T10[])
        n167 = call "Datalog - Queue Driver.vi"("Cases"=RT-_Queue_States."Enqueue Priority", "error in (no error)"=w316, "Element In"=cluster{"Data":variant, "State":T12} {"Data"=variant, "State"=enum."Close File"}) -> ("error out"=w304:errorcluster)  [unwired: 6 in, 2 out]
        n168 = To Variant(anything=w307) -> (Variant=w306:variant)
        n169 = Bundle By Name(cluster=cluster{"Data":variant, "State":T8} {"Data"=variant, "State"=enum."Test Started"} ("Element In"), "Data"=w306) -> (w305:cluster{"Data":variant, "State":T8})
        n170 = call "TCP - Sender Queue Driver.vi"("Cases"=RT-_Queue_States."Enqueue", "error in (no error)"=w304, "Element In"=w305) -> ()  [unwired: 6 in, 3 out]
      }
      frame "Change Dyno Selection" {
        n171 = Variant To Data(error in=w340, type=variant[] [], Variant=w339) -> (data=w336:variant[], error out=w338:errorcluster)
        n172 = Index Array(array=w336) -> (element #1=w335:variant, element #2=w333:variant)  [unwired: 2 in]
        n173 = Variant To Data(type="", Variant=w335) -> (data=w326:string)  [unwired: 1 in, 1 out]
        n174 = Variant To Data(type=T19 {"proportional gain (Kc)"=0.0, "integral time (Ti, min)"=0.0, "derivative time (Td, min)"=0.0} ("PID gains"), Variant=w333) -> (data=w331:T19)  [unwired: 1 in, 1 out]
        n175 = call "FGV - Dyno Config.vi"("Control"=Dyno_Config_Driver."Write File", "error in (no error)"=w338, "PID gains"=w331, "Dyno"=w326, "Dyno Type"=w326) -> ("error out"=w330:errorcluster)  [unwired: 5 in, 1 out]
        n176 = call "FGV - Dyno Config.vi"("Control"=Dyno_Config_Driver."Read File", "error in (no error)"=w330, "Dyno"=w326, "Dyno Type"=w326) -> ("error out"=w328:errorcluster)  [unwired: 6 in, 1 out]
        n177 = call "FGV - Dyno Config.vi"("Control"=Dyno_Config_Driver."Set", "error in (no error)"=w328, "Dyno"=w326, "Dyno Type"=w326) -> ()  [unwired: 6 in, 2 out]
      }
      frame "Get Dyno Config" {
        n178 = Variant To Data(error in=w360, type="", Variant=w358) -> (data=w344:string, error out=w359:errorcluster)
        n179 = call "FGV - Dyno Config.vi"("Control"=Dyno_Config_Driver."Set", "error in (no error)"=w359, "Dyno"=w344, "Dyno Type"=w344) -> ("error out"=w356:errorcluster)  [unwired: 6 in, 1 out]
        n180 = call "FGV - Dyno Config.vi"("Control"=Dyno_Config_Driver."Get", "error in (no error)"=w356) -> ("error out"=w347:errorcluster, "Dyno Parameters"=w346:T20)  [unwired: 8 in]
        n181 = To Variant(anything=w346) -> (Variant=w345:variant)
        n182 = Bundle By Name(cluster=T10 {"Signal"=enum."Log Path", "Value"=FALSE, "Data"=variant}, "Signal"=TCP_-_Signal_Names."Get PID Values", "Data"=w345) -> (w352:T10)
        n183 = Build Array(w352) -> (w350:T10[])
        n184 = To Variant(anything=w350) -> (Variant=w349:variant)
        n185 = Bundle By Name(cluster=cluster{"Data":variant, "State":T8} {"Data"=variant, "State"=enum."Test Started"} ("Element In"), "Data"=w349) -> (w348:cluster{"Data":variant, "State":T8})
        n186 = call "TCP - Sender Queue Driver.vi"("Cases"=RT-_Queue_States."Enqueue", "error in (no error)"=w347, "Element In"=w348) -> ()  [unwired: 6 in, 3 out]
      }
    }
  }
  "error out" <- "error in (no error)"
